vi "WS1050_AD7747_MeasCAP_Ver1.0.vi"(8 "error in (no error)":errorcluster, 9 "OFFSet Cal":dbl, 10 "AD7747_Number":string="8", 11 "Control":refnum<visa-resource-name>="COM8") -> (0 "error":errorcluster, 1 "CAP (pF)":string, 2 "CAP (pF)":dbl, 3 "Control out":refnum<visa-resource-name>)   [LabVIEW 2012]
panel:
  # "Measure Cap Ad7747"
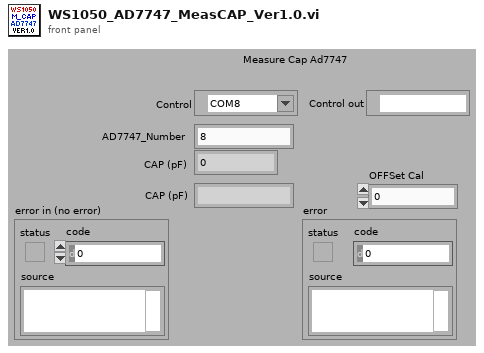
[diagram p1: front panel]
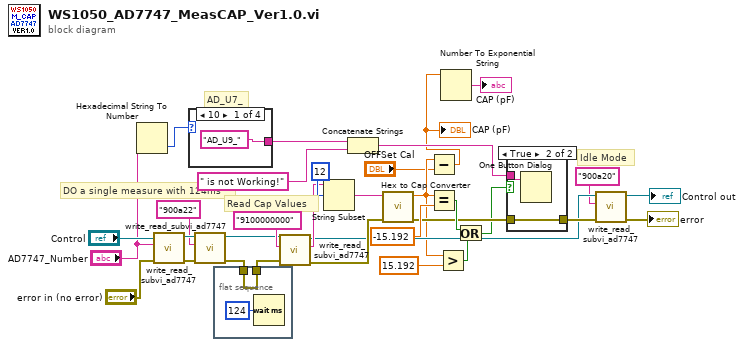
[diagram p0: block diagram]
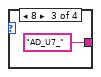
[diagram p3: hidden frame]
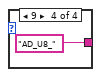
[diagram p4: hidden frame]
diagram:
  # "Idle Mode"
  # "Read Cap Values"
  # "DO a single measure with 124ms"
  # "AD_U7_"
  n1 = Hexadecimal String To Number(string="AD7747_Number") -> (number=w10:u32)  [unwired: 2 in, 1 out]
  n2 = call "write_read_subvi_ad7747.vi"("error in (no error)"="error in (no error)", "command"="AD7747_Number", "Control"="Control") -> ("error out"=w28:errorcluster, "Control out"=w27:refnum<visa-resource-name>)  [unwired: 6 in, 1 out]
  n3 = case shown="10" w10 {
    tunnel: ["AD_U9_" _ "AD_U7_" "AD_U8_"] -> w13
    frame 10 {
    }
    frame 11, Default {
    }
    frame 8 {
    }
    frame 9 {
    }
  }
  n4 = call "write_read_subvi_ad7747.vi"("error in (no error)"=w28, "command"="900a22" ("Data_In 2"), "Control"=w27) -> ("error out"=w18:errorcluster, "Control out"=w26:refnum<visa-resource-name>)  [unwired: 6 in, 1 out]
  n5 = flat-sequence {
    tunnel: w18 -> [w37]
    tunnel: [w37] -> w17
    frame #0 {
      n6 = Wait (ms)(milliseconds to wait=u32 124) -> ()  [unwired: 1 out]
    }
  }
  n7 = call "write_read_subvi_ad7747.vi"("error in (no error)"=w17, "command"="9100000000" ("Data_In 2"), "Control"=w26) -> ("error out"=w32:errorcluster, "output"=w29:string, "Control out"=w7:refnum<visa-resource-name>)  [unwired: 6 in]
  n8 = String Subset(string=w29, offset (0)=12) -> (substring=w30:string)  [unwired: 1 in]
  n9 = Concatenate Strings(w13, " is not Working!" ("Offset Value 2")) -> (w11:string)
  n10 = call "Hex to Cap Converter.vi"(8:w32, "HEX"=w30) -> (0:w20:errorcluster, "CAP (pF)"=w3:dbl)  [unwired: 7 in, 1 out]
  n11 = Subtract(x=w3, y="OFFSet Cal") -> (x-y=w2:dbl)
  "CAP (pF)" <- w2
  n12 = Equal?(x=w3, y=-15.192) -> (x = y?=w22:bool)
  n13 = Greater?(x=w3, y=15.192) -> (0:w21:bool)
  n14 = Number To Exponential String(number=w2) -> (E-format string=→"CAP (pF)":string)  [unwired: 3 in]
  n15 = Or(x=w22, y=w21) -> (x .or. y?=w19:bool)
  n16 = case shown="True" w19 {
    tunnel: w20 -> [w39 w41]
    tunnel: [w39 w41] -> w9
    tunnel: w11 -> [_ w40]
    frame False {
    }
    frame True {
      n17 = One Button Dialog(message=w40) -> ()  [unwired: 1 in, 1 out]
    }
  }
  n18 = call "write_read_subvi_ad7747.vi"("error in (no error)"=w9, "command"="900a20" ("Data_In 2"), "Control"=w7) -> ("error out"=→"error":errorcluster, "Control out"=→"Control out":refnum<visa-resource-name>)  [unwired: 6 in, 1 out]
